vi "Load FP settings from File.vi"(8 "error in":errorcluster) -> (0 "error out":errorcluster)   [LabVIEW 2014, in "POLARIS Vision utility.lvlib"]
uses:
  POLARIS Vision utility.lvlib
  control position.ctl
  <vilib>/Utility/miscctls.llb/LVPositionTypeDef.ctl
  <vilib>/Utility/miscctls.llb/LVBoundsTypeDef.ctl
  <vilib>/Utility/xml.llb/Read From XML File(string).vi
panel:
  in  "Array":T1[](array[typedef])
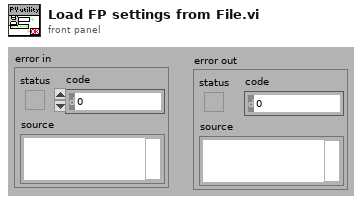
[diagram p1: front panel]
types:
  T1 = typedef "control position.ctl" = cluster{"ControlName":string, "Position":T2, "Size":T3}
  T2 = typedef "LVPositionTypeDef.ctl" = cluster{"Left":i32, "Top":i32}
  T3 = typedef "LVBoundsTypeDef.ctl" = cluster{"Width":u32, "Height":u32}
  T4 = enum32{"invalid app kind", "Development System", "Run Time System", "Student Edition", "Embedded LabVIEW", "Evaluation", "Custom"}
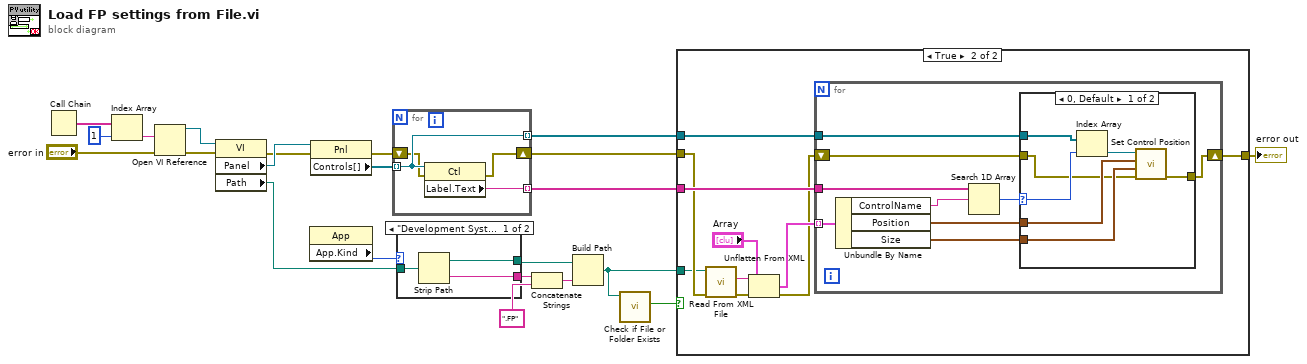
[diagram p0: block diagram]
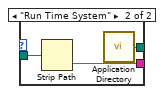
[diagram p4: hidden frame]
diagram:
  n1 = Call Chain() -> (call chain=w19:string[])
  n2 = Index Array(array=w19, index=1) -> (element=w22:string)
  n3 = Open VI Reference(vi path=w22, error in (no error)="error in") -> (vi reference=w17:refnum<vi>, error out=w18:errorcluster)  [unwired: 4 in]
  n4 = property class="VI"(reference=w17, error in=w18) -> (error out=w15:errorcluster, "Panel"=w16:refnum<vi>, "Path"=w13:path)  [unwired: 1 out]
  n5 = property class="App"() -> ("App.Kind"=w12:T4)  [unwired: 2 in, 2 out]
  n6 = property class="Pnl"(reference=w16, error in=w15) -> (error out=w5:errorcluster, "Controls[]"=w14:refnum<vi>[])  [unwired: 1 out]
  n7 = for {
    tunnel: w14 -> [w25] mode=indexing
    tunnel: [w26] -> w7 mode=indexing
    tunnel: [w25] -> w6 mode=indexing
    shift-right: [w23] -> w4
    shift-left: w5 -> [w24]
    n8 = property class="Ctl"(reference=w25, error in=w24) -> (error out=w23:errorcluster, "Label.Text"=w26:string)  [unwired: 1 out]
  }
  n9 = case shown="\"Development System\", Default" w12 {
    tunnel: w13 -> [w29 w32]
    tunnel: [w28 w31] -> w8
    tunnel: [w27 w30] -> w10
    frame "Development System", Default {
      n10 = Strip Path(path=w29) -> (stripped path=w28:path, name=w27:string)
    }
    frame "Run Time System" {
      n11 = Strip Path(path=w32) -> (name=w30:string)  [unwired: 1 out]
      n12 = call <vilib>:"Application Directory.vi"() -> ("Application Directory"=w31:path)
    }
  }
  n13 = Concatenate Strings(w10, ".FP" ("string")) -> (w9:string)
  n14 = Build Path(base path=w8, name or relative path=w9) -> (appended path=w2:path)
  n15 = call <vilib>:"Check if File or Folder Exists.vi"("path"=w2) -> ("file or folder exists?"=w1:bool)  [unwired: 8 in, 2 out]
  n16 = case shown="True" w1 {
    tunnel: w7 -> [_ w40]
    tunnel: w6 -> [_ w39]
    tunnel: w4 -> [w33 w38]
    tunnel: [w33 w35] -> w3
    tunnel: w2 -> [_ w34]
    frame False {
    }
    frame True {
      n17 = call-poly <vilib>:"Read From XML File.vi"("error in (no error)"=w38, "XML File Path"=w34) -> ("error out"=w37:errorcluster, "XML Elements"=w43:string)  [unwired: 7 in, 1 out]
      n18 = Unflatten From XML(xml string=w43, type="Array", error in (no error)=w37) -> (value=w41:T1[], error out=w36:errorcluster)
      n19 = for {
        tunnel: w41 -> [w52] mode=indexing
        tunnel: w40 -> [w51]
        tunnel: w39 -> [w48]
        shift-right: [w44] -> w35
        shift-left: w36 -> [w45]
        n20 = Unbundle By Name(w52) -> ("ControlName"=w50:string, "Position"=w47:T2, "Size"=w46:T3)
        n21 = Search 1D Array(1D array=w51, element=w50) -> (index of element=w49:i32)  [unwired: 1 in]
        n22 = case shown="0, Default" w49 {
          selector: w49 -> [w58 _]
          tunnel: w48 -> [w59 _]
          tunnel: w47 -> [w56 _]
          tunnel: w46 -> [w55 _]
          tunnel: w45 -> [w54 w60]
          tunnel: [w53 w60] -> w44
          frame 0, Default {
            n23 = Index Array(array=w59, index=w58) -> (element=w57:refnum<vi>)
            n24 = call "Set Control Position.vi"("error in (no error)"=w54, "Size"=w55, "Position"=w56, "Ctl Refnum"=w57) -> ("error out"=w53:errorcluster)  [unwired: 5 in, 2 out]
          }
          frame -1 {
          }
        }
      }
    }
  }
  "error out" <- w3
